vi "GetTimeZoneInfo.vi"(8 "error in":errorcluster, 11 "TimeZoneInfoId":string) -> (0 "error out":errorcluster, 2 "OffsetSuffix":string, 3 "Offset":dbl)   [LabVIEW 2021, in "ProligentXMLGenerator.lvlib"]
uses:
  ProligentXMLGenerator.lvlib
  <vilib>/regexp/Match Regular Expression.xnode
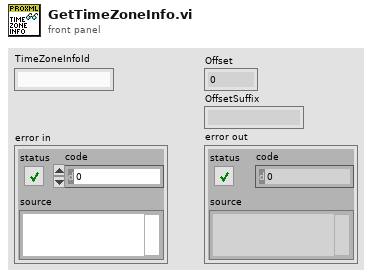
[diagram p1: front panel]
types:
  T1 = enum16{"Native", "Native Command Line", "UNIX", "Macintosh", "DOS"}
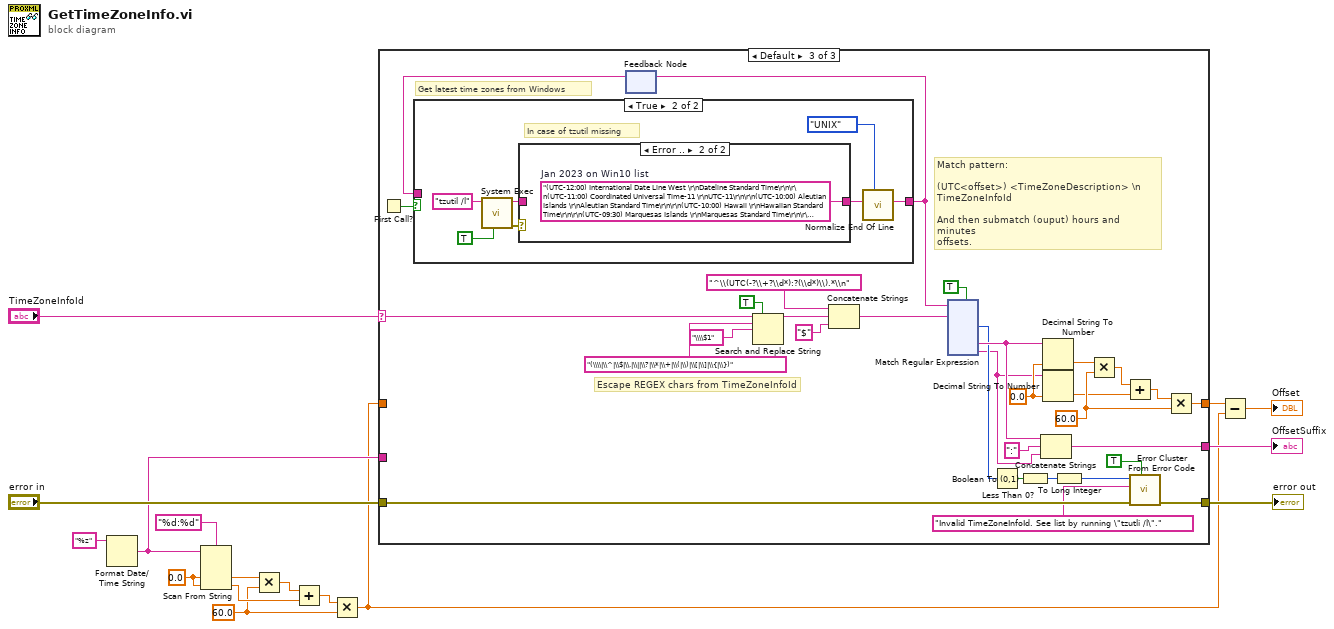
[diagram p0: block diagram]
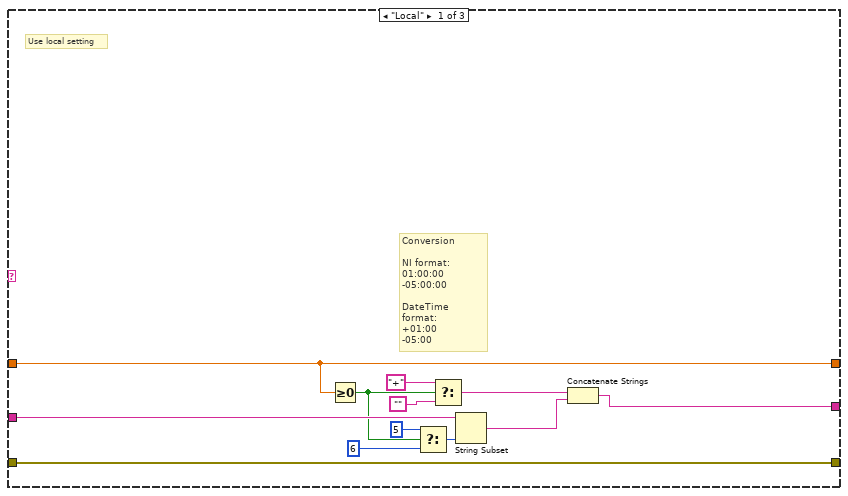
[diagram p2: hidden frame]
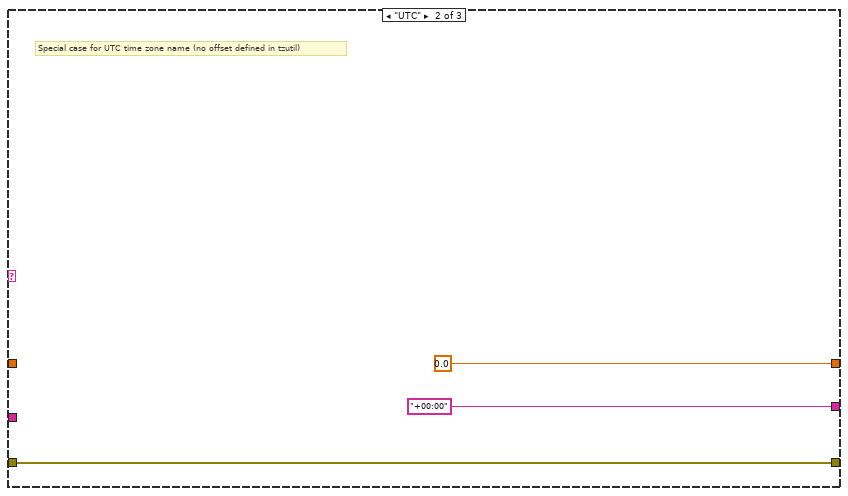
[diagram p3: hidden frame]
diagram:
  w7 = 60.0
  w6 = 0.0
  n1 = Format Date/Time String(time format string (%c)="%z") -> (date/time string=w2:string)  [unwired: 2 in]
  n2 = Scan From String(format string="%d:%d", input string=w2, default 1=w6, default 2=w6) -> (output 1=w10:dbl, output 2=w11:dbl)  [unwired: 2 in, 3 out]
  n3 = Multiply(x=w10, y=w7) -> (x*y=w9:dbl)
  n4 = Add(x=w9, y=w11) -> (x+y=w8:dbl)
  n5 = Multiply(x=w8, y=w7) -> (x*y=w1:dbl)
  n6 = case shown="Default" "TimeZoneInfoId" {
    selector: "TimeZoneInfoId" -> [_ _ w60]
    tunnel: [w28 w29 w62] -> w16
    tunnel: [w18 "+00:00" w61] -> w15
    tunnel: [w27 0.0 w59] -> w12
    tunnel: "error in" -> [w28 w29 w57]
    tunnel: w2 -> [w24 _ _]
    tunnel: w1 -> [w27 _ _]
    frame "Local" {
      # "Conversion\n\nNI format:\n01:00:00\n-05:00:00\n\nDateTime format:\n+01:00\n-05:00"
      # "Use local setting"
      n7 = Greater Or Equal To 0?(x=w27) -> (x >= 0?=w23:bool)
      n8 = Select(t=5, s=w23, f=6 ("length (rest)")) -> (s? t:f=w21:i32)
      n9 = Select(t="+", s=w23, f="") -> (s? t:f=w25:string)
      n10 = String Subset(string=w24, length (rest)=w21) -> (substring=w17:string)  [unwired: 1 in]
      n11 = Concatenate Strings(w25, w17) -> (w18:string)
    }
    frame "UTC" {
      # "Special case for UTC time zone name (no offset defined in tzutil)"
    }
    frame Default {
      w47 = 60.0
      w42 = 0.0
      # "Match pattern:\n\n(UTC<offset>) <TimeZoneDescription> \\n\nTimeZoneInfoId\n\nAnd then submatch (ouput) hours and minutes\noffsets."
      # "Escape REGEX chars from TimeZoneInfoId"
      # "Get latest time zones from Windows"
      n12 = First Call?() -> (First Call?: T/F=w52:bool)
      n13 = feedback #1() -> (w51:string)  [unwired: 1 in]
      n14 = case shown="True" w52 {
        tunnel: [w63 w65] -> w50
        tunnel: w51 -> [w63 _]
        frame False {
        }
        frame True {
          # "In case of tzutil missing"
          n15 = call <vilib>:"System Exec.vi"("run minimized? (F)"=TRUE, "command line"="tzutil /l") -> ("error out"=w68:errorcluster, "standard output"=w67:string)  [unwired: 6 in, 2 out]
          n16 = case shown="Error .." w68 {
            tunnel: w67 -> [w71 _]
            tunnel: [w71 w72] -> w66
            frame No Error {
            }
            frame Error {
              w72 = "(UTC-12:00) International Date Line West \r\nDateline Standard Time\r\n\r\n(UTC-11:00) Coordinated Universal Time-11 \r\nUTC-11\r\n\r\n(UTC-10:00) Aleutian Islands \r\nAleutian Standard Time\r\n\r\n(UTC-10:00) Hawaii \r\nHawaiian Standard Time\r\n\r\n(UTC-09:30) Marquesas Islands \r\nMarquesas Standard Time\r\n\r\n(UTC-09:00) Alaska \r\nAlaskan Standard Time\r\n\r\n(UTC-09:00) Coordinated Universal Time-09 \r\nUTC-09\r\n\r\n(UTC-08:00) Baja California \r\nPacific Standard Time (Mexico)\r\n\r\n(UTC-08:00) Coordinated Universal Time-08 \r\nUTC-08\r\n\r\n(UTC-08:00) Pacific Time (US & Canada) \r\nPacific Standard Time\r\n\r\n(UTC-07:00) Arizona \r\nUS Mountain Standard Time\r\n\r\n(UTC-07:00) Chihuahua, La Paz, Mazatlan \r\nMountain Standard Time (Mexico)\r\n\r\n(UTC-07:00) Mountain Time (US & Canada) \r\nMountain Standard Time\r\n\r\n(UTC-07:00) Yukon \r\nYukon Standard Time\r\n\r\n(UTC-06:00) Central America \r\nCentral America Standard Time\r\n\r\n(UTC-06:00) Central Time (US & Canada) \r\nCentral Standard Time\r\n\r\n(UTC-06:00) Easter Island \r\nEaster Island Standard Time\r\n\r\n(UTC-06:00) Guadalajara, Mexico City, Monterrey \r\nCentral Standard Time (Mexico)\r\n\r\n(UTC-06:00) Saskatchewan \r\nCanada Central Standard Time\r\n\r\n(UTC-05:00) Bogota, Lima, Quito, Rio Branco \r\nSA Pacific Standard Time\r\n\r\n(UTC-05:00) Chetumal \r\nEastern Standard Time (Mexico)\r\n\r\n(UTC-05:00) Eastern Time (US & Canada) \r\nEastern Standard Time\r\n\r\n(UTC-05:00) Haiti \r\nHaiti Standard Time\r\n\r\n(UTC-05:00) Havana \r\nCuba Standard Time\r\n\r\n(UTC-05:00) Indiana (East) \r\nUS Eastern Standard Time\r\n\r\n(UTC-05:00) Turks and Caicos \r\nTurks And Caicos Standard Time\r\n\r\n(UTC-04:00) Asuncion \r\nParaguay Standard Time\r\n\r\n(UTC-04:00) Atlantic Time (Canada) \r\nAtlantic Standard Time\r\n\r\n(UTC-04:00) Caracas \r\nVenezuela Standard Time\r\n\r\n(UTC-04:00) Cuiaba \r\nCentral Brazilian Standard Time\r\n\r\n(UTC-04:00) Georgetown, La Paz, Manaus, San Juan \r\nSA Western Standard Time\r\n\r\n(UTC-04:00) Santiago \r\nPacific SA Standard Time\r\n\r\n(UTC-03:30) Newfoundland \r\nNewfoundland Standard Time\r\n\r\n(UTC-03:00) Araguaina \r\nTocantins Standard Time\r\n\r\n(UTC-03:00) Brasilia \r\nE. South America Standard Time\r\n\r\n(UTC-03:00) Cayenne, Fortaleza \r\nSA Eastern Standard Time\r\n\r\n(UTC-03:00) City of Buenos Aires \r\nArgentina Standard Time\r\n\r\n(UTC-03:00) Greenland \r\nGreenland Standard Time\r\n\r\n(UTC-03:00) Montevideo \r\nMontevideo Standard Time\r\n\r\n(UTC-03:00) Punta Arenas \r\nMagallanes Standard Time\r\n\r\n(UTC-03:00) Saint Pierre and Miquelon \r\nSaint Pierre Standard Time\r\n\r\n(UTC-03:00) Salvador \r\nBahia Standard Time\r\n\r\n(UTC-02:00) Coordinated Universal Time-02 \r\nUTC-02\r\n\r\n(UTC-01:00) Azores \r\nAzores Standard Time\r\n\r\n(UTC-01:00) Cabo Verde Is. \r\nCape Verde Standard Time\r\n\r\n(UTC) Coordinated Universal Time \r\nUTC\r\n\r\n(UTC+00:00) Dublin, Edinburgh, Lisbon, London \r\nGMT Standard Time\r\n\r\n(UTC+00:00) Monrovia, Reykjavik \r\nGreenwich Standard Time\r\n\r\n(UTC+00:00) Sao Tome \r\nSao Tome Standard Time\r\n\r\n(UTC+01:00) Casablanca \r\nMorocco Standard Time\r\n\r\n(UTC+01:00) Amsterdam, Berlin, Bern, Rome, Stockholm, Vienna \r\nW. Europe Standard Time\r\n\r\n(UTC+01:00) Belgrade, Bratislava, Budapest, Ljubljana, Prague \r\nCentral Europe Standard Time\r\n\r\n(UTC+01:00) Brussels, Copenhagen, Madrid, Paris \r\nRomance Standard Time\r\n\r\n(UTC+01:00) Sarajevo, Skopje, Warsaw, Zagreb \r\nCentral European Standard Time\r\n\r\n(UTC+01:00) West Central Africa \r\nW. Central Africa Standard Time\r\n\r\n(UTC+02:00) Athens, Bucharest \r\nGTB Standard Time\r\n\r\n(UTC+02:00) Beirut \r\nMiddle East Standard Time\r\n\r\n(UTC+02:00) Cairo \r\nEgypt Standard Time\r\n\r\n(UTC+02:00) Chisinau \r\nE. Europe Standard Time\r\n\r\n(UTC+02:00) Damascus \r\nSyria Standard Time\r\n\r\n(UTC+02:00) Gaza, Hebron \r\nWest Bank Standard Time\r\n\r\n(UTC+02:00) Harare, Pretoria \r\nSouth Africa Standard Time\r\n\r\n(UTC+02:00) Helsinki, Kyiv, Riga, Sofia, Tallinn, Vilnius \r\nFLE Standard Time\r\n\r\n(UTC+02:00) Jerusalem \r\nIsrael Standard Time\r\n\r\n(UTC+02:00) Juba \r\nSouth Sudan Standard Time\r\n\r\n(UTC+02:00) Kaliningrad \r\nKaliningrad Standard Time\r\n\r\n(UTC+02:00) Khartoum \r\nSudan Standard Time\r\n\r\n(UTC+02:00) Tripoli \r\nLibya Standard Time\r\n\r\n(UTC+02:00) Windhoek \r\nNamibia Standard Time\r\n\r\n(UTC+03:00) Amman \r\nJordan Standard Time\r\n\r\n(UTC+03:00) Baghdad \r\nArabic Standard Time\r\n\r\n(UTC+03:00) Istanbul \r\nTurkey Standard Time\r\n\r\n(UTC+03:00) Kuwait, Riyadh \r\nArab Standard Time\r\n\r\n(UTC+03:00) Minsk \r\nBelarus Standard Time\r\n\r\n(UTC+03:00) Moscow, St. Petersburg \r\nRussian Standard Time\r\n\r\n(UTC+03:00) Nairobi \r\nE. Africa Standard Time\r\n\r\n(UTC+03:00) Volgograd \r\nVolgograd Standard Time\r\n\r\n(UTC+03:30) Tehran \r\nIran Standard Time\r\n\r\n(UTC+04:00) Abu Dhabi, Muscat \r\nArabian Standard Time\r\n\r\n(UTC+04:00) Astrakhan, Ulyanovsk \r\nAstrakhan Standard Time\r\n\r\n(UTC+04:00) Baku \r\nAzerbaijan Standard Time\r\n\r\n(UTC+04:00) Izhevsk, Samara \r\nRussia Time Zone 3\r\n\r\n(UTC+04:00) Port Louis \r\nMauritius Standard Time\r\n\r\n(UTC+04:00) Saratov \r\nSaratov Standard Time\r\n\r\n(UTC+04:00) Tbilisi \r\nGeorgian Standard Time\r\n\r\n(UTC+04:00) Yerevan \r\nCaucasus Standard Time\r\n\r\n(UTC+04:30) Kabul \r\nAfghanistan Standard Time\r\n\r\n(UTC+05:00) Ashgabat, Tashkent \r\nWest Asia Standard Time\r\n\r\n(UTC+05:00) Ekaterinburg \r\nEkaterinburg Standard Time\r\n\r\n(UTC+05:00) Islamabad, Karachi \r\nPakistan Standard Time\r\n\r\n(UTC+05:00) Qyzylorda \r\nQyzylorda Standard Time\r\n\r\n(UTC+05:30) Chennai, Kolkata, Mumbai, New Delhi \r\nIndia Standard Time\r\n\r\n(UTC+05:30) Sri Jayawardenepura \r\nSri Lanka Standard Time\r\n\r\n(UTC+05:45) Kathmandu \r\nNepal Standard Time\r\n\r\n(UTC+06:00) Astana \r\nCentral Asia Standard Time\r\n\r\n(UTC+06:00) Dhaka \r\nBangladesh Standard Time\r\n\r\n(UTC+06:00) Omsk \r\nOmsk Standard Time\r\n\r\n(UTC+06:30) Yangon (Rangoon) \r\nMyanmar Standard Time\r\n\r\n(UTC+07:00) Bangkok, Hanoi, Jakarta \r\nSE Asia Standard Time\r\n\r\n(UTC+07:00) Barnaul, Gorno-Altaysk \r\nAltai Standard Time\r\n\r\n(UTC+07:00) Hovd \r\nW. Mongolia Standard Time\r\n\r\n(UTC+07:00) Krasnoyarsk \r\nNorth Asia Standard Time\r\n\r\n(UTC+07:00) Novosibirsk \r\nN. Central Asia Standard Time\r\n\r\n(UTC+07:00) Tomsk \r\nTomsk Standard Time\r\n\r\n(UTC+08:00) Beijing, Chongqing, Hong Kong, Urumqi \r\nChina Standard Time\r\n\r\n(UTC+08:00) Irkutsk \r\nNorth Asia East Standard Time\r\n\r\n(UTC+08:00) Kuala Lumpur, Singapore \r\nSingapore Standard Time\r\n\r\n(UTC+08:00) Perth \r\nW. Australia Standard Time\r\n\r\n(UTC+08:00) Taipei \r\nTaipei Standard Time\r\n\r\n(UTC+08:00) Ulaanbaatar \r\nUlaanbaatar Standard Time\r\n\r\n(UTC+08:45) Eucla \r\nAus Central W. Standard Time\r\n\r\n(UTC+09:00) Chita \r\nTransbaikal Standard Time\r\n\r\n(UTC+09:00) Osaka, Sapporo, Tokyo \r\nTokyo Standard Time\r\n\r\n(UTC+09:00) Pyongyang \r\nNorth Korea Standard Time\r\n\r\n(UTC+09:00) Seoul \r\nKorea Standard Time\r\n\r\n(UTC+09:00) Yakutsk \r\nYakutsk Standard Time\r\n\r\n(UTC+09:30) Adelaide \r\nCen. Australia Standard Time\r\n\r\n(UTC+09:30) Darwin \r\nAUS Central Standard Time\r\n\r\n(UTC+10:00) Brisbane \r\nE. Australia Standard Time\r\n\r\n(UTC+10:00) Canberra, Melbourne, Sydney \r\nAUS Eastern Standard Time\r\n\r\n(UTC+10:00) Guam, Port Moresby \r\nWest Pacific Standard Time\r\n\r\n(UTC+10:00) Hobart \r\nTasmania Standard Time\r\n\r\n(UTC+10:00) Vladivostok \r\nVladivostok Standard Time\r\n\r\n(UTC+10:30) Lord Howe Island \r\nLord Howe Standard Time\r\n\r\n(UTC+11:00) Bougainville Island \r\nBougainville Standard Time\r\n\r\n(UTC+11:00) Chokurdakh \r\nRussia Time Zone 10\r\n\r\n(UTC+11:00) Magadan \r\nMagadan Standard Time\r\n\r\n(UTC+11:00) Norfolk Island \r\nNorfolk Standard Time\r\n\r\n(UTC+11:00) Sakhalin \r\nSakhalin Standard Time\r\n\r\n(UTC+11:00) Solomon Is., New Caledonia \r\nCentral Pacific Standard Time\r\n\r\n(UTC+12:00) Anadyr, Petropavlovsk-Kamchatsky \r\nRussia Time Zone 11\r\n\r\n(UTC+12:00) Auckland, Wellington \r\nNew Zealand Standard Time\r\n\r\n(UTC+12:00) Coordinated Universal Time+12 \r\nUTC+12\r\n\r\n(UTC+12:00) Fiji \r\nFiji Standard Time\r\n\r\n(UTC+12:45) Chatham Islands \r\nChatham Islands Standard Time\r\n\r\n(UTC+13:00) Coordinated Universal Time+13 \r\nUTC+13\r\n\r\n(UTC+13:00) Nuku'alofa \r\nTonga Standard Time\r\n\r\n(UTC+13:00) Samoa \r\nSamoa Standard Time\r\n\r\n(UTC+14:00) Kiritimati Island \r\nLine Islands Standard Time\r\n\r\n"  # Jan 2023 on Win10 list
            }
          }
          n17 = call <vilib>:"Normalize End Of Line.vi"("end of line (Native)"=T1."UNIX", "string in"=w66) -> ("string out"=w65:string)  [unwired: 6 in]
        }
      }
      n18 = feedback-in #1(w50) -> ()
      n19 = Search and Replace String(replace all?=TRUE ("replace all? (F)"), input string=w60, search string="(\\\\|\\^|\\$|\\.|\\||\\?|\\*|\\+|\\(|\\)|\\[|\\]|\\{|\\})", replace string="\\\\$1" ("replace string (\"\")")) -> (result string=w55:string)  [unwired: 4 in, 3 out]
      n20 = Concatenate Strings("^\\(UTC(-?\\+?\\d*):?(\\d*)\\).*\\n", w55, "$") -> (w37:string)
      n21 = xnode "Match Regular Expression"("input string"=w50, "regular expression"=w37, "multiline? (F)"=TRUE) -> ("offset past match"=w39:i32, "submatch 1"=w49:string, "submatch 2"=w35:string)  [unwired: 3 in, 4 out]
      n22 = Less Than 0?(x=w39) -> (x < 0?=w40:bool)
      n23 = Boolean To (0,1)(Boolean=w40) -> (0, 1=w41:i16)
      n24 = Concatenate Strings(w49, ":" ("string"), w35) -> (w61:string)
      n25 = Decimal String To Number(string=w49, default (0L)=w42) -> (number=w43:dbl)  [unwired: 1 in, 1 out]
      n26 = Decimal String To Number(string=w35, default (0L)=w42) -> (number=w45:dbl)  [unwired: 1 in, 1 out]
      n27 = To Long Integer(number=w41) -> (32bit integer=w56:i32)
      n28 = Multiply(x=w43, y=w47) -> (x*y=w44:dbl)
      n29 = Add(x=w44, y=w45) -> (x+y=w46:dbl)
      n30 = call <vilib>:"Error Cluster From Error Code.vi"("show call chain? (False)"=TRUE, "error in (no error)"=w57, "error message (\"\")"="Invalid TimeZoneInfoId. See list by running \"tzutli /l\"." ("string"), "error code (0)"=w56) -> ("error out"=w62:errorcluster)  [unwired: 5 in]
      n31 = Multiply(x=w46, y=w47) -> (x*y=w59:dbl)
    }
  }
  "error out" <- w16
  "OffsetSuffix" <- w15
  n32 = Subtract(x=w12, y=w1) -> (x-y=→"Offset":dbl)
